vi "Sample Out.vi"(8 "error in (no error)":errorcluster, 11 "Transfer Line in":refnum<class "Transfer Line.lvclass">) -> (0 "error out":errorcluster, 3 "Transfer Line out":refnum<class "Transfer Line.lvclass">)   [LabVIEW 2015, in "cRIO-Carbondioxide.lvlib" / "CO2-Actor.lvlib" / "Transfer Line.lvclass"]
uses:
  Transfer Line.lvclass
  <vilib>/ActorFramework/Message Enqueuer/Message Enqueuer.lvclass/Message Enqueuer.ctl
  <vilib>/ActorFramework/Message Enqueuer/Enqueue.vi
  <vilib>/ActorFramework/Message Priority Queue/Priority Enqueue.vi
  CO2 Actor/CO2 Actor.lvclass
  Transfer Line Messages/Sample Out Msg/Sample Out Msg.lvclass
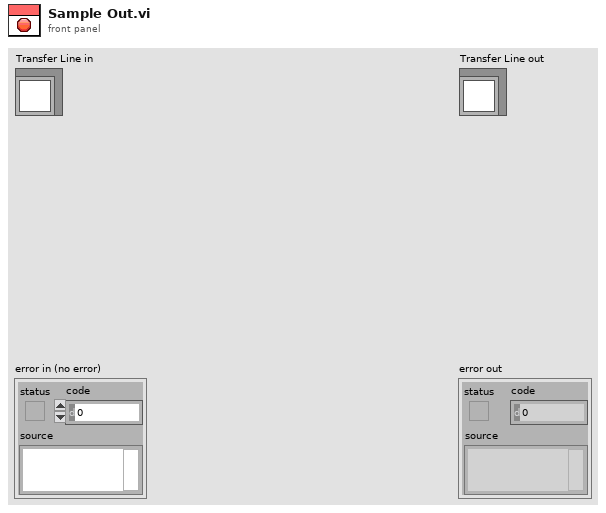
[diagram p1: front panel]
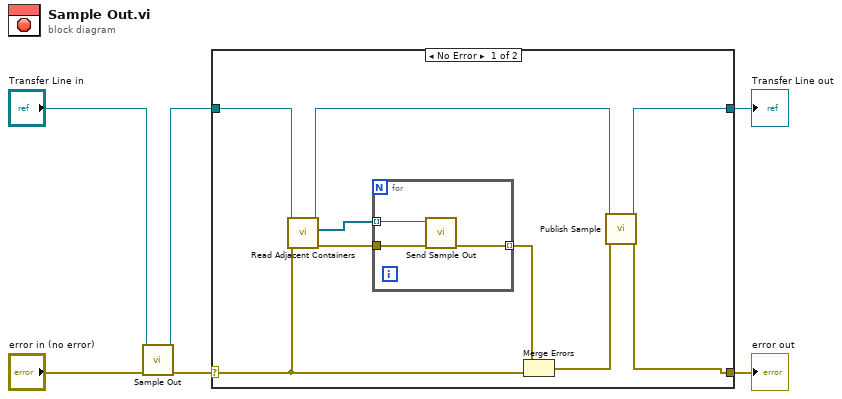
[diagram p0: block diagram]
diagram:
  n1 = call-parent "Sample Out.vi"("error in (no error)"="error in (no error)", "CO2 Actor in"="Transfer Line in") -> ("error out"=w3:errorcluster, "CO2 Actor out"=w1:refnum<class "Transfer Line.lvclass">)  [unwired: 8 in]
  n2 = case shown="No Error" w3 {
    selector: w3 -> [w11 w20]
    tunnel: [w9 w20] -> w6
    tunnel: [w7 w19] -> w5
    tunnel: w1 -> [w12 w19]
    frame No Error {
      n3 = call "Read Adjacent Containers.vi"("error in (no error)"=w11, "Transfer Line in"=w12) -> ("error out"=w15:errorcluster, "Adjacent Containers"=w14:refnum<class "Message Enqueuer.lvclass">[], "Transfer Line out"=w8:refnum<class "Transfer Line.lvclass">)  [unwired: 7 in]
      n4 = for {
        tunnel: w15 -> [w18]
        tunnel: w14 -> [w17] mode=indexing
        tunnel: [w16] -> w13 mode=indexing
        n5 = call "Send Sample Out.vi"("error in (no error)"=w18, "Message Enqueuer"=w17) -> ("error out"=w16:errorcluster)  [unwired: 8 in, 1 out]
      }
      n6 = Merge Errors(w13, w11) -> (w10:errorcluster)
      n7 = call-dynamic "Publish Sample.vi"("error in (no error)"=w10, "Transfer Line in"=w8) -> ("error out"=w9:errorcluster, "Transfer Line out"=w7:refnum<class "Transfer Line.lvclass">)  [unwired: 8 in]
    }
    frame Error {
    }
  }
  "error out" <- w6
  "Transfer Line out" <- w5
